vi "列表框隔行变换颜色.vi"() -> ()   [LabVIEW 2015]
panel:
  in  "stop":bool
  in  "Listbox":i32(listbox)
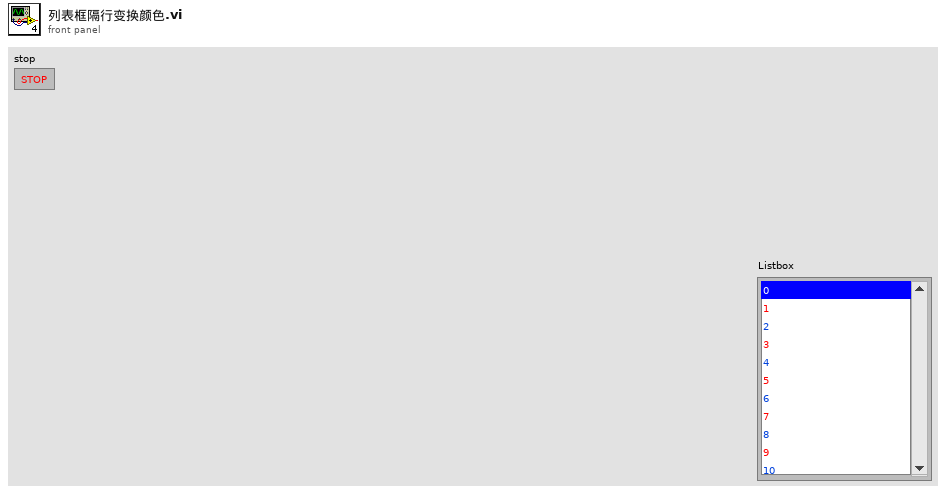
[diagram p1: front panel]
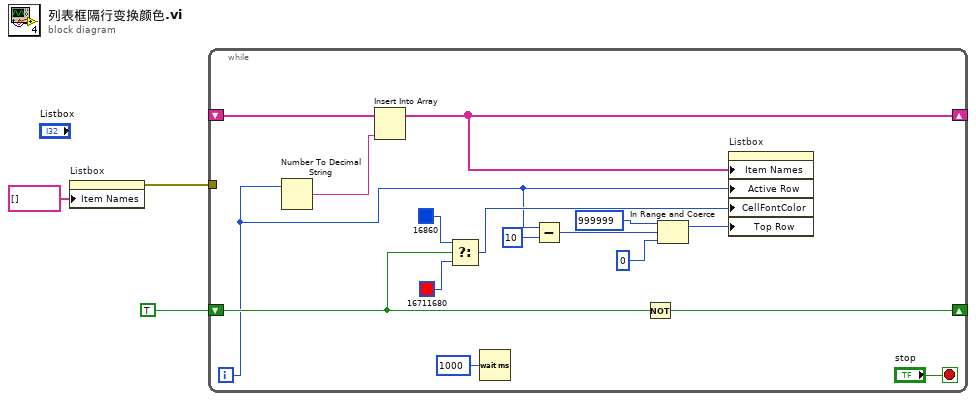
[diagram p0: block diagram]
diagram:
  n1 = property on="Listbox" class="LstBox (strict)"("Item Names"=string[] []) -> (error out=w2:errorcluster)  [unwired: 2 in, 1 out]
  n2 = while {
    tunnel: w2 -> [_]
    shift-right: [w17] -> _
    shift-left: _ -> [w18]
    shift-right: [w16] -> _
    shift-left: TRUE -> [w15]
    i -> [w9]
    stop <- "stop" stop-if-true
    n3 = Number To Decimal String(number=w9) -> (decimal integer string=w19:string)  [unwired: 1 in]
    n4 = Insert Into Array(array=w18, new element=w19) -> (w17:string[])  [unwired: 1 in]
    n5 = Select(t=u32 16860, s=w15, f=u32 16711680) -> (s? t:f=w12:u32)
    n6 = Wait (ms)(milliseconds to wait=u32 1000) -> ()  [unwired: 1 out]
    n7 = Subtract(x=w9, y=10) -> (x-y=w7:i32)
    n8 = Not(x=w15) -> (.not. x?=w16:bool)
    n9 = In Range and Coerce(upper limit=999999, x=w7, lower limit=0) -> (coerced(x)=w6:i32)  [unwired: 1 out]
    n10 = property on="Listbox" class="LstBox (strict)"("Item Names"=w17, "Active Row"=w9, "CellFontColor"=w12, "Top Row"=w6) -> ()  [unwired: 2 in, 2 out]
  }
